vi "Manual Catapult Mode.vi"() -> (14 "high 1":bool, 15 "high 2":bool, 16 "high 3":bool, 17 "high 4":bool, 18 "Jank Boi":bool, 19 "Ball Security":bool)   [LabVIEW 2015]
uses:
  Common Code/Catapult/Catapult Manual Commands.ctl
  Common Code/Change Detect Int.vi
  Robot Global Data.vi
panel:
  out "Finished?":bool
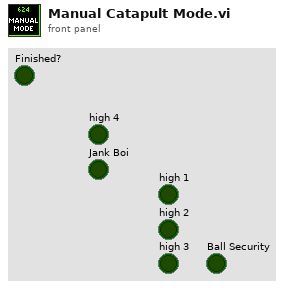
[diagram p1: front panel]
types:
  T1 = typedef "Catapult Manual Commands.ctl" = enum16{"Ready", "Release ", "Shoot"}
  T2 = typedef "Dashboard Control Data.ctl" = cluster{"Shooter Presets":T3, "Encoder Control":T5, "Steer PID output":cluster{"output high":dbl, "output low":dbl}, " Steer PID gains":cluster{"proportional gain (Kc)":dbl, "integral time (Ti, min)":dbl, "derivative time (Td, min)":dbl}, "Drivetrain Settings":T6, "Vision Packet":T7, "Dashboard Drivetrain Command":T8, "Info/Command Cluster":T10, "Ball Vision Packet":T11, "Intake Presets":T13, "Intake Encoder Control":T15, "Climb Presets":T16, "Goal Output Range":cluster{"output high":dbl, "output low":dbl}, "Enabled Systems":T17, "Auton Presets":T18, "Pressure M":dbl, "Pressure B":dbl, "Vision Timeout":dbl, "Auto-Shift":T19, "Catapult Setpoints":T20}
  T3 = typedef "Shooter Presets.ctl" = cluster{"Batter Shot":T4, "Deep Middle":T4, "Manual Shot":T4, "Left Ticks Per Rotation":dbl, "Right Ticks Per Rotation":dbl, "Low Bar Shot":T4, "Shooter RPM Tolerance":dbl, "Trigger Power":dbl, "Fire from Load Delay":i32, "Max Angle":dbl, "Min Angle":dbl, "Angle PID gains":cluster{"P":dbl, "I":dbl, "D":dbl}, "Angle Output":cluster{"output high":dbl, "output low":dbl}, "Shooter Angle Tolerance":dbl, "Vision Shoot x^2":dbl, "Vision Shoot x":dbl, "Feed Forward Max Accel":dbl, "Feed Forward Kv":dbl, "Backwards Trigger":dbl, "Shot Finish Delay (ms)":dbl, "Angle Max Current":dbl, "Angle Current Trip Time":dbl, "Intake Angle":dbl, "Vision Shoot c":dbl, "Reset?":bool, "Button Release Delay":dbl, "Angle Pot x":dbl, "Angle Pot c":dbl, "Ignore Angle?":bool, "Max RPM":dbl, "Safty Frist Angle":dbl, "Intake Danger Height":dbl, "Angle Pot B":i32, "Angle Pot M":dbl, "FF Finish RPM":dbl, "RPM PID Right":cluster{"P":dbl, "I":dbl, "D":dbl, "FF":dbl}, "RPM PID Left":cluster{"P":dbl, "I":dbl, "D":dbl, "FF":dbl}, "Backwards RPM":dbl, "Vision RPM":dbl, "Run Wheels Backward Delay":u32, "Cleat Shot":T4, "Vision Far RPM":dbl, "Vision Far Distance":dbl, "Vision Far Angle":dbl}
  T4 = typedef "Shot Presets.ctl" = cluster{"L":dbl, "R":dbl, "A":dbl}
  T5 = typedef "Encoder Control.ctl" = cluster{"Right Tick Constant":dbl, "Left Tick Constant":dbl, "Reset?":bool, "Y Dist":cluster{"PID gains":cluster{"proportional gain (Kc)":dbl, "integral time (Ti, min)":dbl, "derivative time (Td, min)":dbl}}, "Y Stop Thresh":dbl, "Y Stop Speed":dbl}
  T6 = typedef "Drivetrain Settings.ctl" = cluster{"Gyro Tolerance":dbl, "Throttle Ramp (ms)":dbl, "Kv":dbl, "Ka":dbl, "Feed Forward P":dbl, "Feed Forward D":dbl, "Goal Vision PID gains":cluster{"proportional gain (Kc)":dbl, "integral time (Ti, min)":dbl, "derivative time (Td, min)":dbl}, "Goal Detection Window":dbl, "Creep Rate":dbl, "Vision Throttle Threshold":dbl, "Min Turn Output":dbl, "Left Batter Angle":dbl, "Right Batter Angle":dbl}
  T7 = typedef "Goal Vision Packet.ctl" = cluster{"Distance":dbl, "Center X":dbl, "Center Y":dbl, "Found Target?":bool, "Robot Center":dbl, "Angle":dbl}
  T8 = typedef "Dashboard Drivetrain Command.ctl" = cluster{"Drivetrain Vision":T9}
  T9 = typedef "Drivetrain Vision.ctl" = cluster{"Goal Window":dbl, "Ball Window":dbl}
  T10 = typedef "Ball Tracking Command Cluster.ctl" = cluster{"Distance to Ball":dbl, "Desired Angle":dbl, "Command":enum16{"Turn to Ball", "Turn to Angle", "Get Distance"}, "Pixels from Center":dbl}
  T11 = typedef "Ball Vision Packet.ctl" = cluster{"Ball Detected?":bool, "Distance to Ball":dbl, "Desired Angle":dbl, "Pixels from Center":dbl, "Tracking mode":T12}
  T12 = typedef "Tracking Mode.ctl" = enum16{"Turn to Ball", "Turn to Angle"}
  T13 = typedef "Intake Presets.ctl" = cluster{"Intake Speed":dbl, "Outake Speed":dbl, "Low Height":dbl, "Half Height":dbl, "High Idle Height":dbl, "Angle Speed":dbl, "Angle Tolerance":dbl, "Encoder Scale":dbl, "Load Height":dbl, "Output Range":T14, "Rotation Power Max/Min":dbl, "MaxCurrent":dbl, "Intake Trip Time":dbl, "Idle Height":dbl, "Max Height":dbl, "Reset Encoders?":bool, "PID gains":cluster{"proportional gain (Kc)":dbl, "integral time (Ti, min)":dbl, "derivative time (Td, min)":dbl}, "Intake Stop Delay":u32, "Settle Time":dbl, "Settle Wait Time":dbl, "Pull Up Delay":dbl}
  T14 = typedef "Drivetrain Output Range.ctl" = cluster{"output high":dbl, "output low":dbl}
  T15 = typedef "IntakeEcoderControl.ctl" = cluster{"Arm Tick Constant":dbl, "Reset?":bool, "Y Dist":cluster{"PID gains":cluster{"proportional gain (Kc)":dbl, "integral time (Ti, min)":dbl, "derivative time (Td, min)":dbl}}, "Y Stop Thresh":dbl, "Y Stop Speed":dbl}
  T16 = typedef "Climb Presets.ctl" = cluster{"Pull Power":dbl, "Extend Power":dbl}
  T17 = typedef "Enabled Systems.ctl" = cluster{"Shoot":bool, "Intake":bool, "DT":bool, "Gyro":bool, "100ms":bool, "US":bool}
  T18 = typedef "Autonomous Presets.ctl" = cluster{"Pitch Limit":dbl, "Roll Limit":dbl, "Start Position":dbl, "Cross Position":dbl}
  T19 = typedef "Auto Shift Cluster.ctl" = cluster{"Delay":dbl, "Speed Thresh":dbl, "Upshift Accel":dbl, "Upshift Throttle":dbl, "Upshift Throttle Accel":dbl, "Downshift Throttle":dbl, "Downshift Throttle Accel":dbl, "Pressure Threshold":dbl}
  T20 = typedef "Catapult Presets.ctl" = cluster{"Intake Danger Height":dbl, "Ball Security Delay ":dbl, "PSI Limit":dbl, "Shot Finish Delay":dbl}
  T21 = typedef "Catapult Command Cluster.ctl" = cluster{"Auto Commands":T22, "Mode":T23, "Override IR":bool, "Shoot Mode":T24, "Shoot?":bool, "Manual Commands":T1, "Ball Loaded?":bool, "Batter Ready?":bool}
  T22 = typedef "Catapult Auto Commands.ctl" = enum16{"Idle", "Warmup", "Shoot"}
  T23 = typedef "Shoot Modes Enum.ctl" = enum16{"Manual", "Auto"}
  T24 = typedef "Shoot Mode.ctl" = enum16{"Outer", "Batter"}
  T25 = typedef "Intake Status Cluster.ctl" = cluster{"Roller Power":dbl, "Angle Power":dbl, "Intake Mode":T26, "Intake States":T27, "Rollers Active?":bool, "Current Height":dbl, "Target Height":dbl, "Encoder Raw Position":dbl, "Forward Tripped?":bool, "Backward Tripped?":bool, "Override IR?":bool}
  T26 = typedef "Intake Mode.ctl" = enum16{"Safe", "Auto", "Manual"}
  T27 = typedef "Intake States.ctl" = enum16{"Idle", "Set roller speed", "Move to angle", "Go Hard or Go Home", "Ball Settle"}
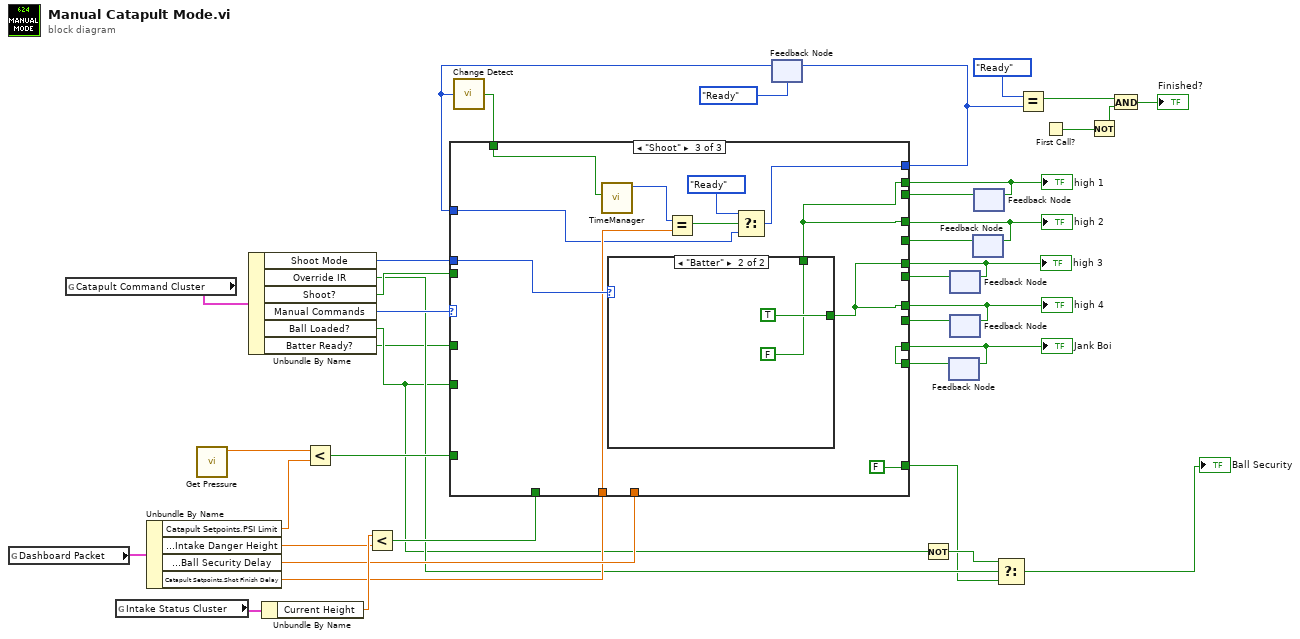
[diagram p0: block diagram]
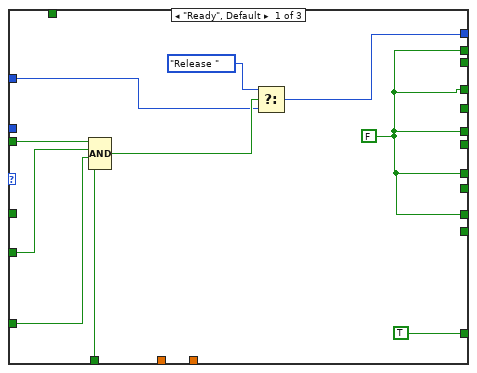
[diagram p2: hidden frame]
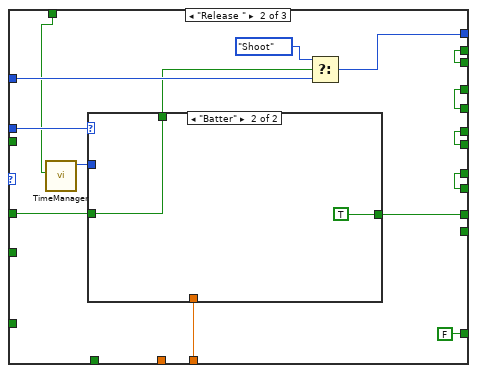
[diagram p3: hidden frame]
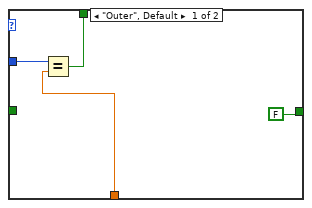
[diagram p4: hidden frame]
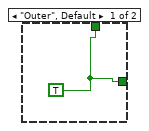
[diagram p5: hidden frame]
diagram:
  n1 = global read "Robot Global Data.vi" "Dashboard Packet"() -> (w36:T2)
  n2 = global read "Robot Global Data.vi" "Catapult Command Cluster"() -> (w39:T21)
  n3 = global read "Robot Global Data.vi" "Intake Status Cluster"() -> (w37:T25)
  n4 = Unbundle By Name(w36) -> ("Catapult Setpoints.PSI Limit"=w34:dbl, "Catapult Setpoints.Intake Danger Height"=w30:dbl, "Catapult Setpoints.Ball Security Delay"=w14:dbl, "Catapult Setpoints.Shot Finish Delay"=w13:dbl)
  n5 = call "Get Pressure.vi"() -> ("Pressure"=w33:dbl)  [unwired: 10 in, 1 out]
  n6 = Unbundle By Name(w39) -> ("Shoot Mode"=w26:T24, "Override IR"=w12:bool, "Shoot?"=w35:bool, "Manual Commands"=w38:T1, "Ball Loaded?"=w2:bool, "Batter Ready?"=w1:bool)
  n7 = Unbundle By Name(w37) -> ("Current Height"=w31:dbl)
  n8 = Less?(x=w33, y=w34) -> (x < y?=w32:bool)
  n9 = Less?(x=w31, y=w30) -> (x < y?=w29:bool)
  n10 = feedback #1(Catapult_Manual_Commands."Ready" ("Manual Commands")) -> (w27:T1)
  n11 = call-poly "Change Detect.vi"("In"=w27) -> ("Changed?"=w15:bool)
  n12 = Not(x=w2) -> (.not. x?=w11:bool)
  n13 = feedback #2() -> (w16:bool)  [unwired: 1 in]
  n14 = feedback #3() -> (w22:bool)  [unwired: 1 in]
  n15 = feedback #4() -> (w24:bool)  [unwired: 1 in]
  n16 = feedback #5() -> (w20:bool)  [unwired: 1 in]
  n17 = feedback #6() -> (w18:bool)  [unwired: 1 in]
  n18 = case shown="\"Shoot\"" w38 {
    tunnel: w35 -> [w49 _ _]
    tunnel: w2 -> [w48 _ _]
    tunnel: w32 -> [w47 _ _]
    tunnel: w29 -> [w46 _ _]
    tunnel: w27 -> [w43 w57 w74]
    tunnel: [w42 w56 w73] -> w7
    tunnel: [w41 w59 w71] -> w19
    tunnel: [w41 w60 w71] -> w21
    tunnel: [w41 w61 w81] -> w23
    tunnel: [w41 w62 w81] -> w25
    tunnel: [w41 w63 w72] -> w17
    tunnel: [TRUE FALSE FALSE] -> w10
    tunnel: w26 -> [_ w64 w82]
    tunnel: w24 -> [_ w62 _]
    tunnel: w22 -> [_ w61 _]
    tunnel: w20 -> [_ w60 _]
    tunnel: w18 -> [_ w59 _]
    tunnel: w16 -> [_ _ w72]
    tunnel: w15 -> [_ w53 w79]
    tunnel: w14 -> [_ w51 _]
    tunnel: w13 -> [_ _ w77]
    tunnel: w1 -> [_ w54 _]
    frame "Ready", Default {
      w41 = FALSE
      n19 = Compound Arithmetic op=AND(w49, w48, w47, w46) -> (w45:bool)
      n20 = Select(t=Catapult_Manual_Commands."Release " ("Manual Commands"), s=w45, f=w43) -> (s? t:f=w42:T1)
    }
    frame "Release " {
      n21 = call "TimeManager.vi"("Reset?"=w53) -> ("Time Since Reset"=w52:u32)  [unwired: 9 in, 1 out]
      n22 = case shown="\"Batter\"" w64 {
        tunnel: [FALSE TRUE] -> w63
        tunnel: w54 -> [_ w69]
        tunnel: w52 -> [w67 _]
        tunnel: w51 -> [w66 _]
        tunnel: [w65 w69] -> w50
        frame "Outer", Default {
          n23 = Equal?(x=w67, y=w66) -> (x = y?=w65:bool)
        }
        frame "Batter" {
        }
      }
      n24 = Select(t=Catapult_Manual_Commands."Shoot" ("Manual Commands"), s=w50, f=w57) -> (s? t:f=w56:T1)
    }
    frame "Shoot" {
      n25 = call "TimeManager.vi"("Reset?"=w79) -> ("Time Since Reset"=w78:u32)  [unwired: 9 in, 1 out]
      n26 = case shown="\"Batter\"" w82 {
        tunnel: [w83 TRUE] -> w81
        tunnel: [w83 FALSE] -> w71
        frame "Outer", Default {
          w83 = TRUE
        }
        frame "Batter" {
        }
      }
      n27 = Equal?(x=w78, y=w77) -> (x = y?=w76:bool)
      n28 = Select(t=Catapult_Manual_Commands."Ready" ("Manual Commands"), s=w76, f=w74) -> (s? t:f=w73:T1)
    }
  }
  "high 1" <- w19
  "high 2" <- w21
  "high 3" <- w23
  "high 4" <- w25
  "Jank Boi" <- w17
  n29 = feedback-in #1(w7) -> ()
  n30 = feedback-in #2(w17) -> ()
  n31 = feedback-in #3(w23) -> ()
  n32 = feedback-in #4(w25) -> ()
  n33 = feedback-in #5(w21) -> ()
  n34 = feedback-in #6(w19) -> ()
  n35 = Select(t=w11, s=w12, f=w10) -> (s? t:f=→"Ball Security":bool)
  n36 = Equal?(x=Catapult_Manual_Commands."Ready" ("Manual Commands"), y=w7) -> (x = y?=w5:bool)
  n37 = First Call?() -> (First Call?: T/F=w8:bool)
  n38 = Not(x=w8) -> (.not. x?=w4:bool)
  n39 = And(x=w5, y=w4) -> (x .and. y?=→"Finished?":bool)
